vi "gyro -- async pll monitor V2.vi"(8 "pll engine pair IN":T7, 11 "pll monitor event pair IN":T7) -> ()   [LabVIEW 2020]
uses:
  agregator -- action.ctl
  four-corner circle transformation.ctl
  cursor action.ctl
  interpolation state - real.ctl
  publisher action.ctl
  pll internal user event action.ctl
  server talkto message type.ctl
  circle corners.ctl
  lorentzian.ctl
  show-win- control.ctl
  <vilib>/event_ctls.llb/eventvkey.ctl
  server talkback message type.ctl
  server talk-to-back pair.ctl
panel:
  in  "all 3":T1(tab)
  in  "Reset lore :q":bool
  in  "Tab Control":enum32{"PID", "hist", "params"}(tab)=enum."params"
  out "Plot: complex plane":cluster{dbl[], dbl[]}[](graph)=[{[1.788783031557316e-06, 1.7433846913024676e-06, 1.607269314653193e-06, 1.380675694232449e-06, 1.0640013522474786e-06, 6.578018431007985e-07, 1.627897787589622e-07, -4.201664214109396e-07, -1.090044054143964e-06, -1.845667926446343e-06, -2.6857124172833478e-06, -3.6087038031690138e-06, -4.613022843577905e-06, -5.6969076216432555e-06, -6.858456635157808e-06, -8.095632132454864e-06, -9.406263687317083e-06, -1.0788052006641661e-05, -1.2238572964181675e-05, -1.375528185328725e-05, -1.5335517851185776e-05, -1.6976508686969115e-05, -1.8675375505098885e-05, -2.0429137915897256e-05, -2.2234719224163222e-05, -2.4088951826741428e-05, -2.5988582769574486e-05, -2.793027945448972e-05, -2.991063548570884e-05, -3.1926176645823585e-05, -3.397336699075361e-05, -3.604861505299396e-05, -3.814828014226944e-05, -4.026867873254248e-05, -4.240609092416943e-05, -4.455676696986866e-05, -4.671693385305138e-05, -4.888280190697483e-05, -5.105057146310552e-05, -5.321643951702898e-05, -5.5376606400211694e-05, -5.752728244591091e-05, -5.9664694637537876e-05, -6.178509322781091e-05, -6.38847583170864e-05, -6.596000637932674e-05, -6.800719672425677e-05, -7.002273788437151e-05, -7.200309391559062e-05, -7.394479060050587e-05, -7.584442154333893e-05, -7.769865414591714e-05, -7.95042354541831e-05, -8.125799786498148e-05, -8.295686468311124e-05, -8.459785551889458e-05, -8.61780915167931e-05, -8.769480040589868e-05, -8.91453213634387e-05, -9.052710968276327e-05, -9.18377412376255e-05, -9.307491673492255e-05, -9.42364657484371e-05, -9.532035052650245e-05, -9.632466956691135e-05, -9.724766095279701e-05, -9.808770544363402e-05, -9.88433293159364e-05, -9.951320694866943e-05, -0.00010009616314883933, -0.00010059117521318116, -0.00010099737472232784, -0.0001013140490643128, -0.00010154064268473356, -0.00010167675806138284, -0.00010172215640163768, -0.00010167675806138284, -0.00010154064268473356, -0.00010131404906431282, -0.00010099737472232786, -0.00010059117521318118, -0.00010009616314883934, -9.951320694866943e-05, -9.88433293159364e-05, -9.808770544363403e-05, -9.724766095279704e-05, -9.632466956691136e-05, -9.532035052650247e-05, -9.423646574843712e-05, -9.307491673492258e-05, -9.183774123762553e-05, -9.05271096827633e-05, -8.914532136343872e-05, -8.769480040589871e-05, -8.617809151679313e-05, -8.459785551889461e-05, -8.295686468311128e-05, -8.12579978649815e-05, -7.950423545418313e-05, -7.769865414591716e-05, -7.584442154333896e-05, -7.39447906005059e-05, -7.200309391559066e-05, -7.002273788437154e-05, -6.80071967242568e-05, -6.596000637932677e-05, -6.388475831708641e-05, -6.178509322781096e-05, -5.966469463753793e-05, -5.752728244591097e-05, -5.5376606400211735e-05, -5.321643951702903e-05, -5.105057146310557e-05, -4.888280190697487e-05, -4.671693385305141e-05, -4.45567669698687e-05, -4.2406090924169466e-05, -4.02686787325425e-05, -3.814828014226947e-05, -3.604861505299398e-05, -3.3973366990753624e-05, -3.192617664582364e-05, -2.9910635485708896e-05, -2.7930279454489773e-05, -2.5988582769574527e-05, -2.4088951826741472e-05, -2.223471922416326e-05, -2.042913791589729e-05, -1.8675375505098912e-05, -1.6976508686969142e-05, -1.5335517851185796e-05, -1.375528185328727e-05, -1.2238572964181688e-05, -1.0788052006641675e-05, -9.406263687317096e-06, -8.09563213245487e-06, -6.858456635157842e-06, -5.696907621643283e-06, -4.613022843577932e-06, -3.608703803169034e-06, -2.685712417283368e-06, -1.8456679264463634e-06, -1.0900440541439775e-06, -4.2016642141095315e-07, 1.6278977875895542e-07, 6.578018431007917e-07, 1.0640013522474786e-06, 1.3806756942324422e-06, 1.607269314653193e-06, 1.7433846913024676e-06], [0.00010355923614313292, 0.00010572653027157724, 0.00010789002222966876, 0.00011004591651735351, 0.00011219043096347307, 0.00011431980336097804, 0.00011643029806711761, 0.00011851821255702628, 0.00012057988391921064, 0.00012261169528154077, 0.00012461008215647302, 0.00012657153869437233, 0.00012849262383396383, 0.00013036996733912354, 0.0001322002757114178, 0.00013398033796801863, 0.00013570703127485878, 0.00013737732642514367, 0.00013898829315360961, 0.00014053710527720475, 0.00014202104565317432, 0.00014343751094585263, 0.0001447840161937981, 0.0001460581991692603, 0.00014725782452233005, 0.00014838078770250255, 0.00014942511865077436, 0.00015038898525579616, 0.00015127069656801869, 0.00015206870576619277, 0.00015278161287101945, 0.00015340816720118942, 0.00015394726956750299, 0.0001543979742012214, 0.0001547594904132666, 0.00015503118398135874, 0.00015521257826265722, 0.00015530335502995444, 0.00015530335502995444, 0.00015521257826265722, 0.00015503118398135874, 0.00015475949041326664, 0.0001543979742012214, 0.00015394726956750299, 0.00015340816720118942, 0.00015278161287101945, 0.00015206870576619277, 0.0001512706965680187, 0.0001503889852557962, 0.00014942511865077439, 0.00014838078770250258, 0.00014725782452233005, 0.00014605819916926034, 0.0001447840161937981, 0.00014343751094585263, 0.00014202104565317434, 0.00014053710527720475, 0.00013898829315360964, 0.0001373773264251437, 0.00013570703127485878, 0.00013398033796801863, 0.00013220027571141782, 0.00013036996733912354, 0.00012849262383396383, 0.00012657153869437236, 0.00012461008215647305, 0.0001226116952815408, 0.00012057988391921064, 0.00011851821255702631, 0.00011643029806711764, 0.00011431980336097807, 0.00011219043096347309, 0.00011004591651735353, 0.00010789002222966877, 0.00010572653027157724, 0.00010355923614313295, 0.00010139194201468863, 9.92284500565971e-05, 9.707255576891236e-05, 9.492804132279279e-05, 9.279866892528782e-05, 9.068817421914825e-05, 8.860025972923959e-05, 8.653858836705524e-05, 8.45067770047251e-05, 8.250839012979284e-05, 8.054693359189351e-05, 7.862584845230203e-05, 7.674850494714233e-05, 7.491819657484808e-05, 7.313813431824723e-05, 7.141144101140709e-05, 6.97411458611222e-05, 6.813017913265623e-05, 6.658136700906111e-05, 6.509742663309153e-05, 6.368096134041324e-05, 6.233445609246777e-05, 6.106027311700553e-05, 5.9860647763935806e-05, 5.87376845837633e-05, 5.769335363549149e-05, 5.6729487030469677e-05, 5.584777571824716e-05, 5.5049766520073076e-05, 5.433685941524639e-05, 5.371030508507641e-05, 5.317120271876287e-05, 5.2720498085044465e-05, 5.235898187299923e-05, 5.2087288304907106e-05, 5.1905894023608635e-05, 5.181511725631141e-05, 5.18151172563114e-05, 5.1905894023608635e-05, 5.20872883049071e-05, 5.2358981872999216e-05, 5.272049808504446e-05, 5.3171202718762854e-05, 5.37103050850764e-05, 5.433685941524638e-05, 5.5049766520073056e-05, 5.584777571824713e-05, 5.672948703046965e-05, 5.769335363549145e-05, 5.8737684583763264e-05, 5.986064776393577e-05, 6.10602731170055e-05, 6.233445609246772e-05, 6.368096134041321e-05, 6.50974266330915e-05, 6.658136700906109e-05, 6.81301791326562e-05, 6.974114586112215e-05, 7.141144101140706e-05, 7.31381343182472e-05, 7.491819657484801e-05, 7.674850494714228e-05, 7.862584845230197e-05, 8.054693359189346e-05, 8.250839012979277e-05, 8.450677700472503e-05, 8.653858836705518e-05, 8.860025972923954e-05, 9.06881742191482e-05, 9.279866892528778e-05, 9.492804132279275e-05, 9.70725557689123e-05, 9.922845005659706e-05, 0.00010139194201468859]}, {[1.679879022748994e-06, -3.4847775480299235e-06, -8.649434118808841e-06, -1.3814090689587757e-05, -1.8978747260366676e-05, -2.4143403831145596e-05, -2.9308060401924508e-05, -3.447271697270343e-05, -3.963737354348235e-05, -4.4802030114261266e-05, -4.9966686685040185e-05, -5.51313432558191e-05, -6.029599982659801e-05, -6.546065639737694e-05, -7.062531296815585e-05, -7.578996953893478e-05, -8.095462610971369e-05, -8.61192826804926e-05, -9.128393925127153e-05, -9.644859582205044e-05], [0.00010691496202238116, 0.00010657938943445635, 0.00010624381684653152, 0.00010590824425860668, 0.00010557267167068187, 0.00010523709908275705, 0.00010490152649483222, 0.00010456595390690739, 0.00010423038131898257, 0.00010389480873105775, 0.00010355923614313292, 0.00010322366355520809, 0.00010288809096728327, 0.00010255251837935846, 0.00010221694579143363, 0.0001018813732035088, 0.00010154580061558398, 0.00010121022802765916, 0.00010087465543973433, 0.0001005390828518095]}, {[-4.6610960805791945e-05, -4.694653339371677e-05, -4.728210598164159e-05, -4.761767856956642e-05, -4.795325115749124e-05, -4.8288823745416065e-05, -4.862439633334089e-05, -4.895996892126571e-05, -4.929554150919054e-05, -4.963111409711536e-05, -4.9966686685040185e-05, -5.0302259272965016e-05, -5.0637831860889833e-05, -5.0973404448814664e-05, -5.130897703673949e-05, -5.164454962466431e-05, -5.1980122212589136e-05, -5.231569480051396e-05, -5.2651267388438784e-05, -5.298683997636361e-05], [5.191267043534376e-05, 5.7077327006122676e-05, 6.22419835769016e-05, 6.740664014768051e-05, 7.257129671845942e-05, 7.773595328923835e-05, 8.290060986001726e-05, 8.806526643079617e-05, 9.322992300157508e-05, 9.839457957235401e-05, 0.00010355923614313292, 0.00010872389271391185, 0.00011388854928469076, 0.00011905320585546967, 0.0001242178624262486, 0.00012938251899702753, 0.00013454717556780644, 0.00013971183213858535, 0.00014487648870936426, 0.00015004114528014318]}, {[8.391330781245461e-06, 7.720185605395813e-06, 7.049040429546165e-06, 6.377895253696517e-06, 5.706750077846869e-06, 5.035604901997221e-06, 4.364459726147573e-06, 3.6933145502979247e-06, 3.0221693744482766e-06, 2.3510241985986286e-06, 1.6798790227489805e-06, 1.0087338468993325e-06, 3.3758867104968446e-07, -3.335565047999636e-07, -1.0047016806496116e-06, -1.6758468564992597e-06, -2.3469920323489077e-06, -3.0181372081985558e-06, -3.689282384048204e-06, -4.360427559897852e-06], [3.6218306068028043e-06, 1.395114374836064e-05, 2.4280456889918475e-05, 3.4609770031476307e-05, 4.4939083173034145e-05, 5.5268396314591984e-05, 6.559770945614981e-05, 7.592702259770765e-05, 8.625633573926549e-05, 9.658564888082332e-05, 0.00010691496202238116, 0.00011724427516393899, 0.0001275735883054968, 0.00013790290144705467, 0.0001482322145886125, 0.00015856152773017034, 0.00016889084087172817, 0.000179220154013286, 0.00018954946715484384, 0.00019987878029640167]}]
  out "Plot: complex- hist":cluster{dbl[], dbl[]}[](graph)=[{array[1000 elements], array[1000 elements]}, {[1.788783031557316e-06, 1.7433846913024676e-06, 1.607269314653193e-06, 1.380675694232449e-06, 1.0640013522474786e-06, 6.578018431007985e-07, 1.627897787589622e-07, -4.201664214109396e-07, -1.090044054143964e-06, -1.845667926446343e-06, -2.6857124172833478e-06, -3.6087038031690138e-06, -4.613022843577905e-06, -5.6969076216432555e-06, -6.858456635157808e-06, -8.095632132454864e-06, -9.406263687317083e-06, -1.0788052006641661e-05, -1.2238572964181675e-05, -1.375528185328725e-05, -1.5335517851185776e-05, -1.6976508686969115e-05, -1.8675375505098885e-05, -2.0429137915897256e-05, -2.2234719224163222e-05, -2.4088951826741428e-05, -2.5988582769574486e-05, -2.793027945448972e-05, -2.991063548570884e-05, -3.1926176645823585e-05, -3.397336699075361e-05, -3.604861505299396e-05, -3.814828014226944e-05, -4.026867873254248e-05, -4.240609092416943e-05, -4.455676696986866e-05, -4.671693385305138e-05, -4.888280190697483e-05, -5.105057146310552e-05, -5.321643951702898e-05, -5.5376606400211694e-05, -5.752728244591091e-05, -5.9664694637537876e-05, -6.178509322781091e-05, -6.38847583170864e-05, -6.596000637932674e-05, -6.800719672425677e-05, -7.002273788437151e-05, -7.200309391559062e-05, -7.394479060050587e-05, -7.584442154333893e-05, -7.769865414591714e-05, -7.95042354541831e-05, -8.125799786498148e-05, -8.295686468311124e-05, -8.459785551889458e-05, -8.61780915167931e-05, -8.769480040589868e-05, -8.91453213634387e-05, -9.052710968276327e-05, -9.18377412376255e-05, -9.307491673492255e-05, -9.42364657484371e-05, -9.532035052650245e-05, -9.632466956691135e-05, -9.724766095279701e-05, -9.808770544363402e-05, -9.88433293159364e-05, -9.951320694866943e-05, -0.00010009616314883933, -0.00010059117521318116, -0.00010099737472232784, -0.0001013140490643128, -0.00010154064268473356, -0.00010167675806138284, -0.00010172215640163768, -0.00010167675806138284, -0.00010154064268473356, -0.00010131404906431282, -0.00010099737472232786, -0.00010059117521318118, -0.00010009616314883934, -9.951320694866943e-05, -9.88433293159364e-05, -9.808770544363403e-05, -9.724766095279704e-05, -9.632466956691136e-05, -9.532035052650247e-05, -9.423646574843712e-05, -9.307491673492258e-05, -9.183774123762553e-05, -9.05271096827633e-05, -8.914532136343872e-05, -8.769480040589871e-05, -8.617809151679313e-05, -8.459785551889461e-05, -8.295686468311128e-05, -8.12579978649815e-05, -7.950423545418313e-05, -7.769865414591716e-05, -7.584442154333896e-05, -7.39447906005059e-05, -7.200309391559066e-05, -7.002273788437154e-05, -6.80071967242568e-05, -6.596000637932677e-05, -6.388475831708641e-05, -6.178509322781096e-05, -5.966469463753793e-05, -5.752728244591097e-05, -5.5376606400211735e-05, -5.321643951702903e-05, -5.105057146310557e-05, -4.888280190697487e-05, -4.671693385305141e-05, -4.45567669698687e-05, -4.2406090924169466e-05, -4.02686787325425e-05, -3.814828014226947e-05, -3.604861505299398e-05, -3.3973366990753624e-05, -3.192617664582364e-05, -2.9910635485708896e-05, -2.7930279454489773e-05, -2.5988582769574527e-05, -2.4088951826741472e-05, -2.223471922416326e-05, -2.042913791589729e-05, -1.8675375505098912e-05, -1.6976508686969142e-05, -1.5335517851185796e-05, -1.375528185328727e-05, -1.2238572964181688e-05, -1.0788052006641675e-05, -9.406263687317096e-06, -8.09563213245487e-06, -6.858456635157842e-06, -5.696907621643283e-06, -4.613022843577932e-06, -3.608703803169034e-06, -2.685712417283368e-06, -1.8456679264463634e-06, -1.0900440541439775e-06, -4.2016642141095315e-07, 1.6278977875895542e-07, 6.578018431007917e-07, 1.0640013522474786e-06, 1.3806756942324422e-06, 1.607269314653193e-06, 1.7433846913024676e-06], [0.00010355923614313292, 0.00010572653027157724, 0.00010789002222966876, 0.00011004591651735351, 0.00011219043096347307, 0.00011431980336097804, 0.00011643029806711761, 0.00011851821255702628, 0.00012057988391921064, 0.00012261169528154077, 0.00012461008215647302, 0.00012657153869437233, 0.00012849262383396383, 0.00013036996733912354, 0.0001322002757114178, 0.00013398033796801863, 0.00013570703127485878, 0.00013737732642514367, 0.00013898829315360961, 0.00014053710527720475, 0.00014202104565317432, 0.00014343751094585263, 0.0001447840161937981, 0.0001460581991692603, 0.00014725782452233005, 0.00014838078770250255, 0.00014942511865077436, 0.00015038898525579616, 0.00015127069656801869, 0.00015206870576619277, 0.00015278161287101945, 0.00015340816720118942, 0.00015394726956750299, 0.0001543979742012214, 0.0001547594904132666, 0.00015503118398135874, 0.00015521257826265722, 0.00015530335502995444, 0.00015530335502995444, 0.00015521257826265722, 0.00015503118398135874, 0.00015475949041326664, 0.0001543979742012214, 0.00015394726956750299, 0.00015340816720118942, 0.00015278161287101945, 0.00015206870576619277, 0.0001512706965680187, 0.0001503889852557962, 0.00014942511865077439, 0.00014838078770250258, 0.00014725782452233005, 0.00014605819916926034, 0.0001447840161937981, 0.00014343751094585263, 0.00014202104565317434, 0.00014053710527720475, 0.00013898829315360964, 0.0001373773264251437, 0.00013570703127485878, 0.00013398033796801863, 0.00013220027571141782, 0.00013036996733912354, 0.00012849262383396383, 0.00012657153869437236, 0.00012461008215647305, 0.0001226116952815408, 0.00012057988391921064, 0.00011851821255702631, 0.00011643029806711764, 0.00011431980336097807, 0.00011219043096347309, 0.00011004591651735353, 0.00010789002222966877, 0.00010572653027157724, 0.00010355923614313295, 0.00010139194201468863, 9.92284500565971e-05, 9.707255576891236e-05, 9.492804132279279e-05, 9.279866892528782e-05, 9.068817421914825e-05, 8.860025972923959e-05, 8.653858836705524e-05, 8.45067770047251e-05, 8.250839012979284e-05, 8.054693359189351e-05, 7.862584845230203e-05, 7.674850494714233e-05, 7.491819657484808e-05, 7.313813431824723e-05, 7.141144101140709e-05, 6.97411458611222e-05, 6.813017913265623e-05, 6.658136700906111e-05, 6.509742663309153e-05, 6.368096134041324e-05, 6.233445609246777e-05, 6.106027311700553e-05, 5.9860647763935806e-05, 5.87376845837633e-05, 5.769335363549149e-05, 5.6729487030469677e-05, 5.584777571824716e-05, 5.5049766520073076e-05, 5.433685941524639e-05, 5.371030508507641e-05, 5.317120271876287e-05, 5.2720498085044465e-05, 5.235898187299923e-05, 5.2087288304907106e-05, 5.1905894023608635e-05, 5.181511725631141e-05, 5.18151172563114e-05, 5.1905894023608635e-05, 5.20872883049071e-05, 5.2358981872999216e-05, 5.272049808504446e-05, 5.3171202718762854e-05, 5.37103050850764e-05, 5.433685941524638e-05, 5.5049766520073056e-05, 5.584777571824713e-05, 5.672948703046965e-05, 5.769335363549145e-05, 5.8737684583763264e-05, 5.986064776393577e-05, 6.10602731170055e-05, 6.233445609246772e-05, 6.368096134041321e-05, 6.50974266330915e-05, 6.658136700906109e-05, 6.81301791326562e-05, 6.974114586112215e-05, 7.141144101140706e-05, 7.31381343182472e-05, 7.491819657484801e-05, 7.674850494714228e-05, 7.862584845230197e-05, 8.054693359189346e-05, 8.250839012979277e-05, 8.450677700472503e-05, 8.653858836705518e-05, 8.860025972923954e-05, 9.06881742191482e-05, 9.279866892528778e-05, 9.492804132279275e-05, 9.70725557689123e-05, 9.922845005659706e-05, 0.00010139194201468859]}, {[1.679879022748994e-06, -3.4847775480299235e-06, -8.649434118808841e-06, -1.3814090689587757e-05, -1.8978747260366676e-05, -2.4143403831145596e-05, -2.9308060401924508e-05, -3.447271697270343e-05, -3.963737354348235e-05, -4.4802030114261266e-05, -4.9966686685040185e-05, -5.51313432558191e-05, -6.029599982659801e-05, -6.546065639737694e-05, -7.062531296815585e-05, -7.578996953893478e-05, -8.095462610971369e-05, -8.61192826804926e-05, -9.128393925127153e-05, -9.644859582205044e-05], [0.00010691496202238116, 0.00010657938943445635, 0.00010624381684653152, 0.00010590824425860668, 0.00010557267167068187, 0.00010523709908275705, 0.00010490152649483222, 0.00010456595390690739, 0.00010423038131898257, 0.00010389480873105775, 0.00010355923614313292, 0.00010322366355520809, 0.00010288809096728327, 0.00010255251837935846, 0.00010221694579143363, 0.0001018813732035088, 0.00010154580061558398, 0.00010121022802765916, 0.00010087465543973433, 0.0001005390828518095]}, {[-4.6610960805791945e-05, -4.694653339371677e-05, -4.728210598164159e-05, -4.761767856956642e-05, -4.795325115749124e-05, -4.8288823745416065e-05, -4.862439633334089e-05, -4.895996892126571e-05, -4.929554150919054e-05, -4.963111409711536e-05, -4.9966686685040185e-05, -5.0302259272965016e-05, -5.0637831860889833e-05, -5.0973404448814664e-05, -5.130897703673949e-05, -5.164454962466431e-05, -5.1980122212589136e-05, -5.231569480051396e-05, -5.2651267388438784e-05, -5.298683997636361e-05], [5.191267043534376e-05, 5.7077327006122676e-05, 6.22419835769016e-05, 6.740664014768051e-05, 7.257129671845942e-05, 7.773595328923835e-05, 8.290060986001726e-05, 8.806526643079617e-05, 9.322992300157508e-05, 9.839457957235401e-05, 0.00010355923614313292, 0.00010872389271391185, 0.00011388854928469076, 0.00011905320585546967, 0.0001242178624262486, 0.00012938251899702753, 0.00013454717556780644, 0.00013971183213858535, 0.00014487648870936426, 0.00015004114528014318]}, {[8.391330781245461e-06, 7.720185605395813e-06, 7.049040429546165e-06, 6.377895253696517e-06, 5.706750077846869e-06, 5.035604901997221e-06, 4.364459726147573e-06, 3.6933145502979247e-06, 3.0221693744482766e-06, 2.3510241985986286e-06, 1.6798790227489805e-06, 1.0087338468993325e-06, 3.3758867104968446e-07, -3.335565047999636e-07, -1.0047016806496116e-06, -1.6758468564992597e-06, -2.3469920323489077e-06, -3.0181372081985558e-06, -3.689282384048204e-06, -4.360427559897852e-06], [3.6218306068028043e-06, 1.395114374836064e-05, 2.4280456889918475e-05, 3.4609770031476307e-05, 4.4939083173034145e-05, 5.5268396314591984e-05, 6.559770945614981e-05, 7.592702259770765e-05, 8.625633573926549e-05, 9.658564888082332e-05, 0.00010691496202238116, 0.00011724427516393899, 0.0001275735883054968, 0.00013790290144705467, 0.0001482322145886125, 0.00015856152773017034, 0.00016889084087172817, 0.000179220154013286, 0.00018954946715484384, 0.00019987878029640167]}, {[nan, nan, nan, nan, nan, nan, nan, nan, nan, nan, nan, nan, nan, nan, nan, nan, nan, nan, nan, nan], [nan, nan, nan, nan, nan, nan, nan, nan, nan, nan, nan, nan, nan, nan, nan, nan, nan, nan, nan, nan]}]
  in  "dt (sec)":dbl=0.001 format="%#_10f"
  in  "plot hist time (sec)":dbl=1.0 format="%#_10f"
  out "G (Hz)":dbl=inf format="%#.4f"
  in  "Reset freq :r":bool
  in  "lorentzian":T2={"A (VHz)"=0.0013462087701026876, "f (Hz)"=46382.17969574165, "G (Hz)"=26.010946813433538, "phi(rad)"=-1.5059127195190136, "Q"=1783.1792140602604, "Norm  Ampl"=nan, "bg (V)"=1.6798790227489873e-06+0.00010691496202238116i, "4corners"={"z (-pi/2)"=-4.6610960805791945e-05+5.191267043534375e-05i, "z(inf)"=1.6798790227489873e-06+0.00010691496202238116i, "z (pi/2)"=-5.332241256428843e-05+0.0001552058018509221i, "z center"=-4.9966686685040185e-05+0.00010355923614313292i, "z(0)"=-0.00010161325239282936+0.00010020351026388468i, "radius"=5.17554697165975e-05}} {"bg (V)" format="%#9_9f"; "Q" format="%#9_9f"; "phi(rad)" format="%#9_9f"; "G (Hz)" format="%#9_9f"; "f (Hz)" format="%#9_9f"}
  in  "Toggle PLL :@":bool
  out "f (Hz)":dbl=6.94898403792542e-310 format="%#.11f"
  in  "PLL is ON":bool
  in  "publish delay":u32=30
  out "VKey":T4=enum."Cmd"
  out "Char":i16
  in  "lorentzian -- basic":T2={"A (VHz)"=1.0, "f (Hz)"=1000.0, "G (Hz)"=3.0, "phi(rad)"=0.0, "Q"=300.0, "Norm  Ampl"=nan, "bg (V)"=0.0+0.0i, "4corners"={"z (-pi/2)"=9.277908004825974e-07+0.0007240755403629966i, "z(inf)"=2.6527949823343002e-05+0.0007477540585896028i, "z (pi/2)"=2.8494315967368497e-06+0.0007733542176124632i, "z center"=1.8886111986097237e-06+0.0007487148789877299i, "z(0)"=-2.2750727426123552e-05+0.000749675699385857i, "radius"=2.4658065287076567e-05}} {"bg (V)" format="%#9_9f"; "Q" format="%#9_9f"; "phi(rad)" format="%#9_9f"; "G (Hz)" format="%#9_9f"; "f (Hz)" format="%#9_9f"}
  in  "save lor for later":bool
  in  "reset from basic":bool
  out "zi out Im (V)":dbl=8e-323 format="%#.8f"
  out "zi out Re (V)":dbl=1e-323 format="%#.8f"
  out "publish message":T5={"freq (Hz)"=6.94898403792542e-310, "gamma (Hz)"=inf, "Voltage (V)"=1e-323+8e-323i}
  out "is publish loop stoped?":bool=TRUE
  out "window":T6={"cen (Hz)"=45496.74569300777, "win (Hz)"=29.962105514646385, "left (Hz)"=45481.76464025045, "right (Hz)"=45511.72674576509}
  in  "lorentzian -- hist":T2={"A (VHz)"=0.0013462087701026876, "f (Hz)"=46382.17969574165, "G (Hz)"=26.010946813433538, "phi(rad)"=-1.5059127195190136, "Q"=1783.1792140602604, "Norm  Ampl"=nan, "bg (V)"=1.6798790227489873e-06+0.00010691496202238116i, "4corners"={"z (-pi/2)"=-4.6610960805791945e-05+5.191267043534375e-05i, "z(inf)"=1.6798790227489873e-06+0.00010691496202238116i, "z (pi/2)"=-5.332241256428843e-05+0.0001552058018509221i, "z center"=-4.9966686685040185e-05+0.00010355923614313292i, "z(0)"=-0.00010161325239282936+0.00010020351026388468i, "radius"=5.17554697165975e-05}} {"bg (V)" format="%#9_9f"; "Q" format="%#9_9f"; "phi(rad)" format="%#9_9f"; "G (Hz)" format="%#9_9f"; "f (Hz)" format="%#9_9f"}
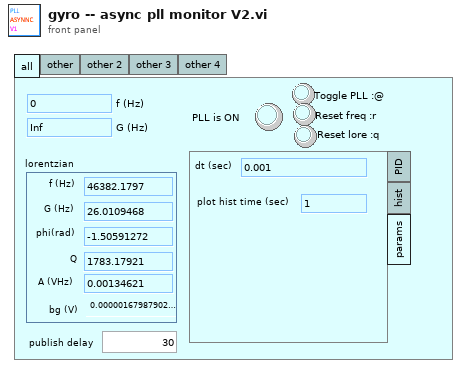
[diagram p1: front panel]
types:
  T1 = enum32{"all", "other", "other 2", "other 3", "other 4"}
  T2 = typedef "lorentzian.ctl" = cluster{"A (VHz)":dbl, "f (Hz)":dbl, "G (Hz)":dbl, "phi(rad)":dbl, "Q":dbl, "Norm  Ampl":dbl, "bg (V)":cdb, "4corners":T3}
  T3 = typedef "circle corners.ctl" = cluster{"z (-pi/2)":cdb, "z(inf)":cdb, "z (pi/2)":cdb, "z center":cdb, "z(0)":cdb, "radius":dbl}
  T4 = typedef "eventvkey.ctl" = enum16{"ASCII", "Enter", "Return", "Shift", "Ctrl", "Alt", "Cmd", "Opt", "Caps", "NumLock", "Clear", "Break", "Up", "Down", "Left", "Right", "Insert", "Delete", "Home", "End", "PageUp", "PageDown", "Escape", "Help", "Pause", "ScrollLock", "F1", "F2", "F3", "F4", "F5", "F6", "F7", "F8", "F9", "F10", "F11", "F12", "F13", "F14", "F15", "F16", "F17", "F18", "F19", "F20", "F21", "F22", "F23", "F24", "Play", "VolumeUp", "VolumeDown", "Mute", "Two Byte Char"}
  T5 = cluster{"freq (Hz)":dbl, "gamma (Hz)":dbl, "Voltage (V)":cdb}
  T6 = typedef "show-win- control.ctl" = cluster{"cen (Hz)":dbl, "win (Hz)":dbl, "left (Hz)":dbl, "right (Hz)":dbl}
  T7 = typedef "server talk-to-back pair.ctl" = cluster{"talkback event":refnum<user-event>, "talkto event":refnum<user-event>}
  T8 = typedef "pll internal user event action.ctl" = enum16{"gear pll engine", "start pll async", "stop pll async", "toggle pll async", "gear sweeper", "start sweeper", "stop sweeper", "toggle sweeper", "accept frequency", "reset lorentzian", "accept lorentzian", "update cursors", "pause pll", "unpause pll", "void", "exit", "gear sweeper monitor", "gear sweeper engine", "gear fitter", "gear sourcer", "gear pll monitor"}
  T9 = typedef "interpolation state - real.ctl" = cluster{"requested size":i32, "Array":dbl[], "actual number of elements":i32}
  T10 = typedef "agregator -- action.ctl" = enum16{"append", "interpolate", "empty!", "force", "init", "scale", "read last"}
  T11 = typedef "publisher action.ctl" = enum16{"set", "get", "init", "check"}
  T12 = typedef "four-corner circle transformation.ctl" = enum16{"z(c) z(inf)", "z(c) z(zero)", "fix phase", "calculate lorentzian", "z(0) z(+-pi/2)", "shift to zcenter", "to  canonical", "get canonical phase", "get4corners", "update lorentzian -- from z0", "fake gamma normal", "fake gamma heat", "calculate complex slope", "get f0 given f and phi"}
  T13 = typedef "interpolation state - complex.ctl" = cluster{"requested size":i32, "Array":cdb[], "actual number of elements":i32}
  T14 = typedef "server talkto message type.ctl" = cluster{"message":enum16{"stop", "start", "update pars", "update request", "new", "launch", "exit", "get", "reset", "pause", "unpause"}}
  T15 = typedef "cursor action.ctl" = enum16{"range", "read", "write", "check", "zoom out", "smart zoom out", "zoom to aspect ratio 1", "zoom to win", "zoom out 20%", "zoom in 20%", "-empty", "smart zoom out&aspect", "move range left 20%", "move range right 20%", "move range up 20%", "move range down 20%", "zoom to X win", "zoom to Y win", "zoom out X", "zoom out Y", "zoom in X", "zoom in Y", "check plot scale"}
  T16 = typedef "pll talkback data type.ctl" = cluster{"freq (Hz)":dbl, "gamma (Hz)":dbl, "Voltage (V)":cdb, "overlimit ?":bool, "running lorentzian out":T2, "static lorentzian out":T2}
  T17 = enum16{"stop", "start", "update pars", "update request", "new", "launch", "exit", "get", "reset", "pause", "unpause"}
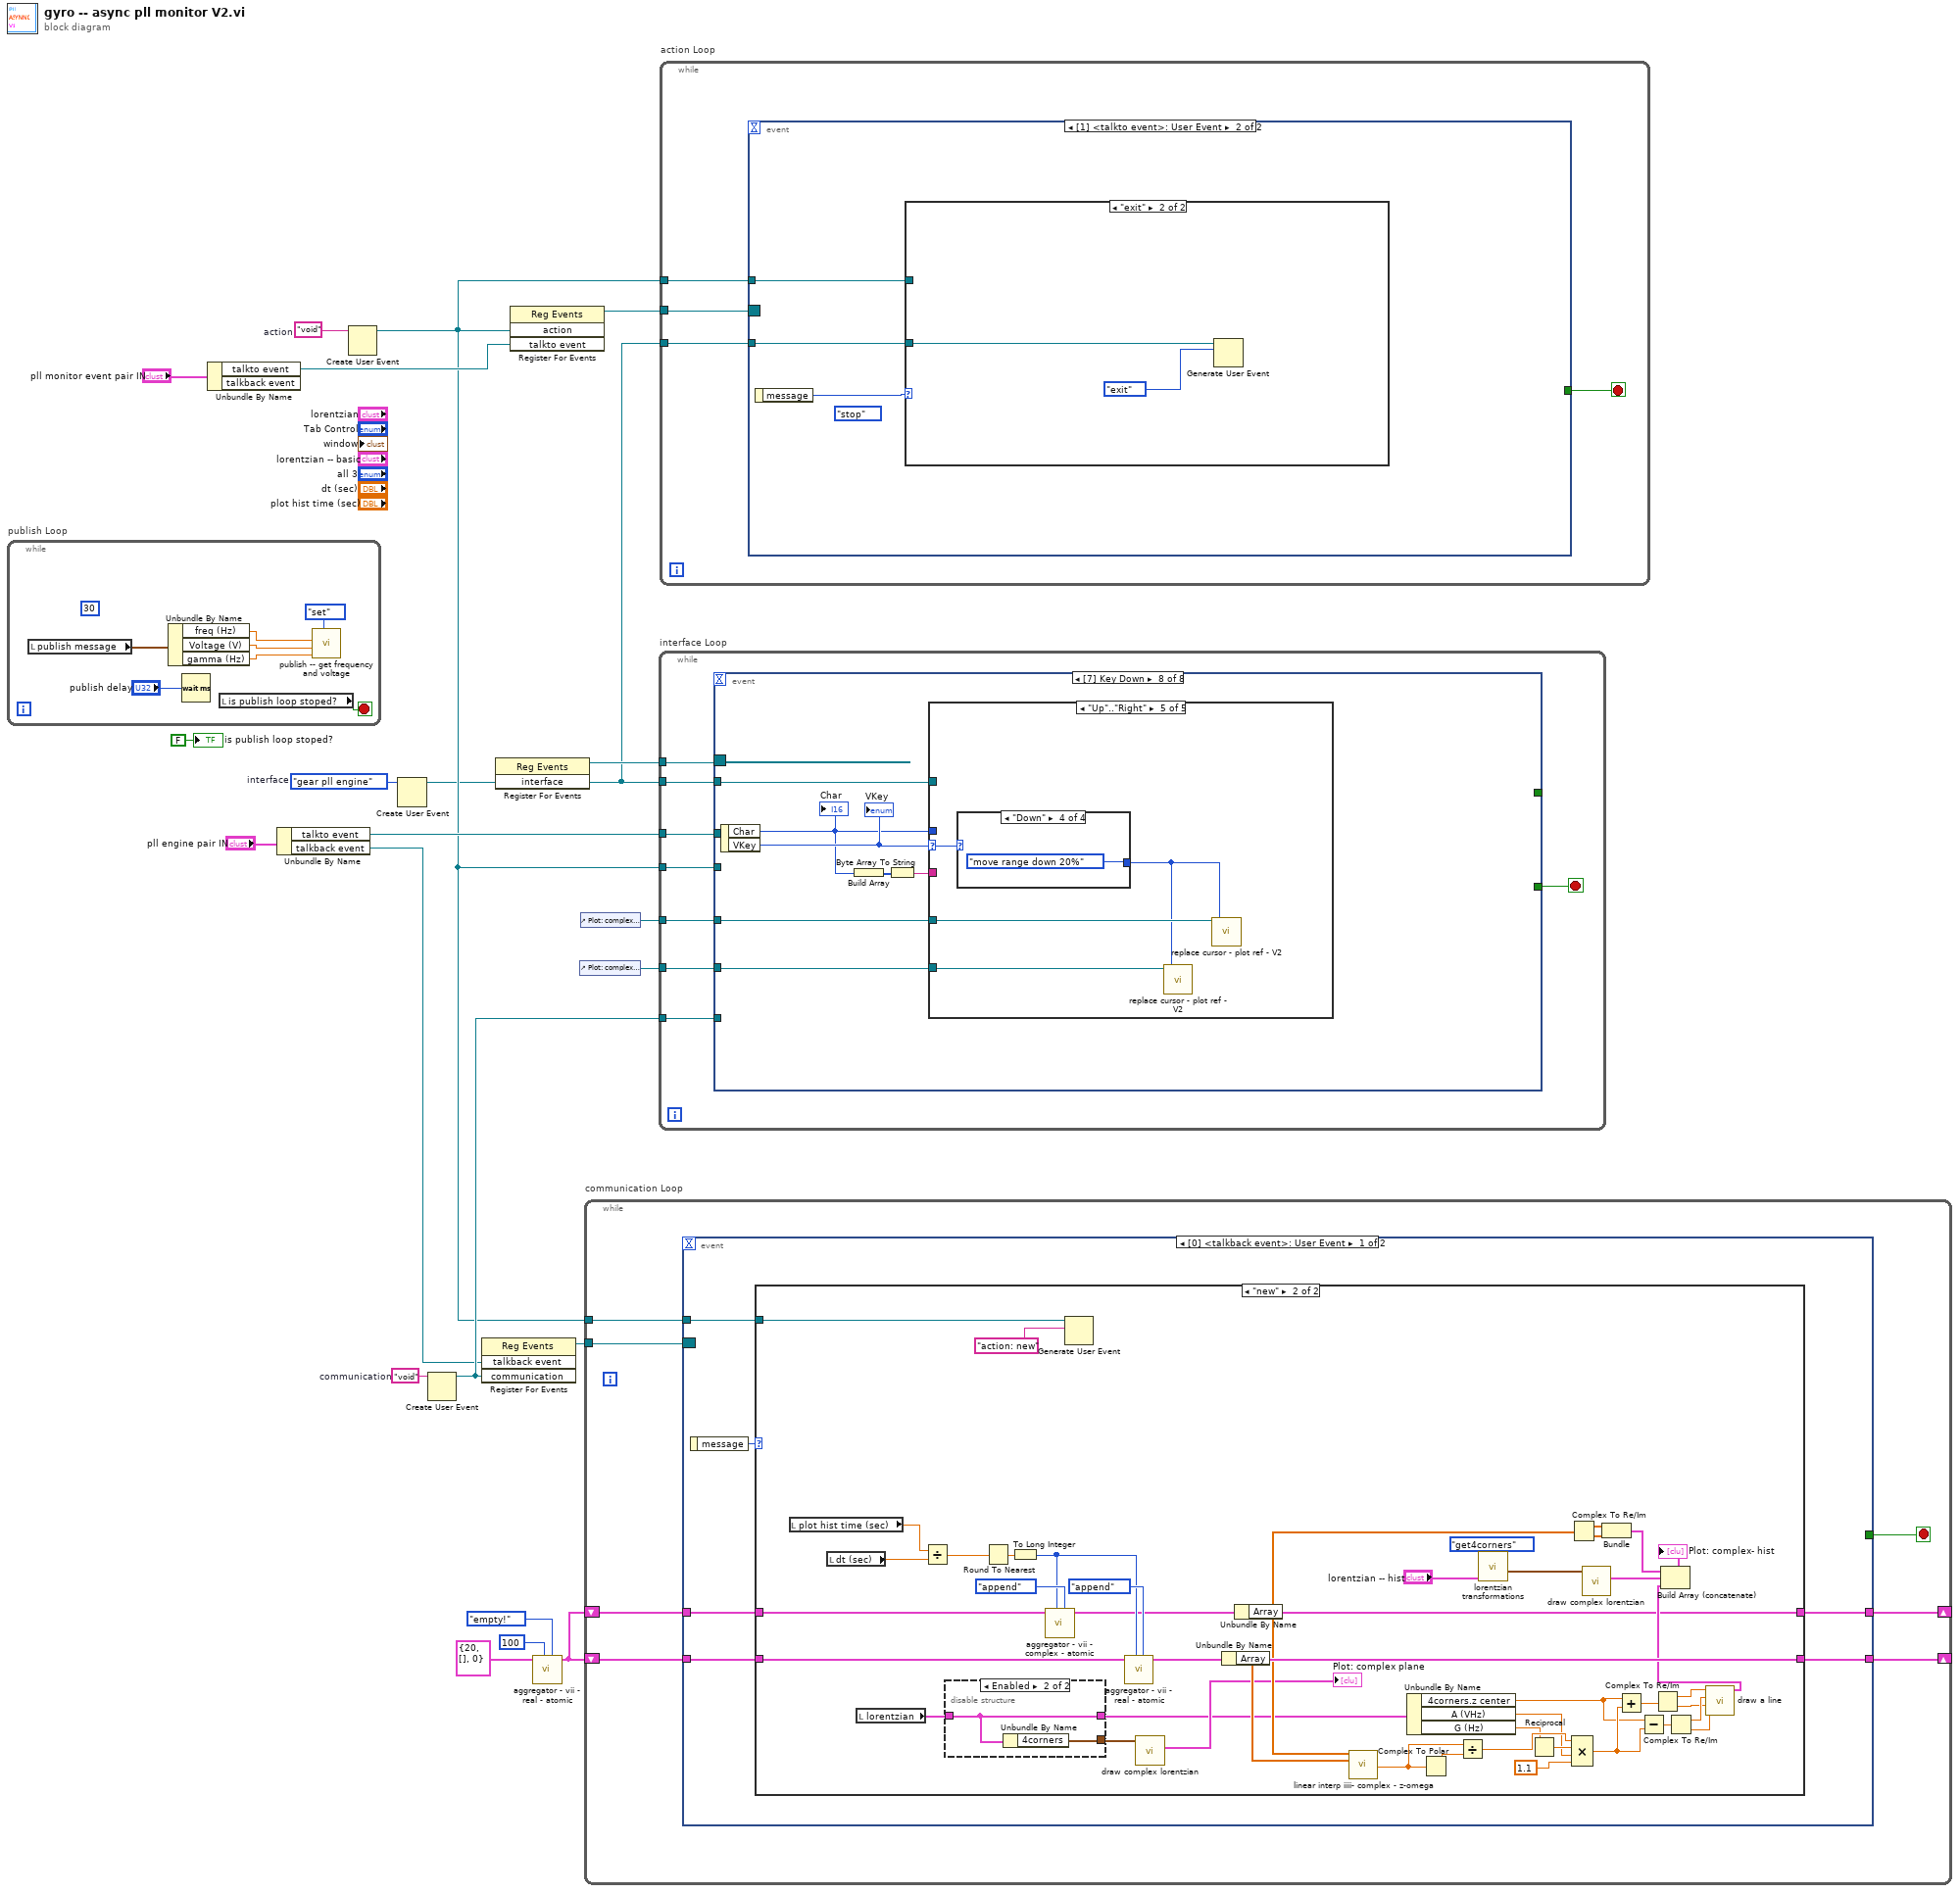
[diagram p0: block diagram]
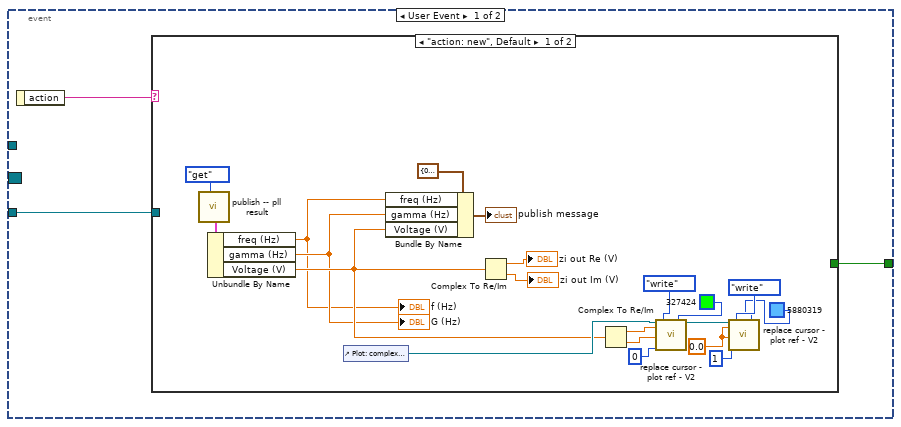
[diagram p2: hidden frame]
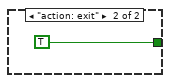
[diagram p3: hidden frame]
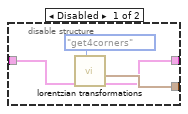
[diagram p6: hidden frame]
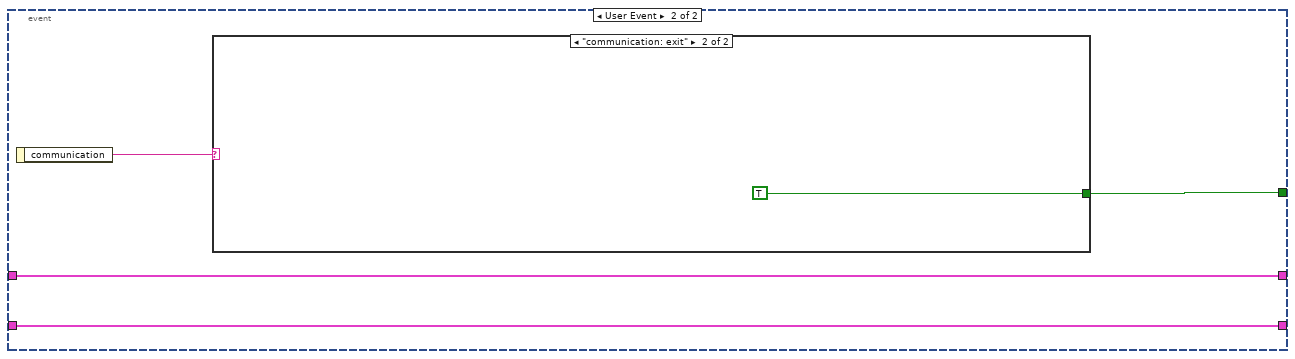
[diagram p7: hidden frame]
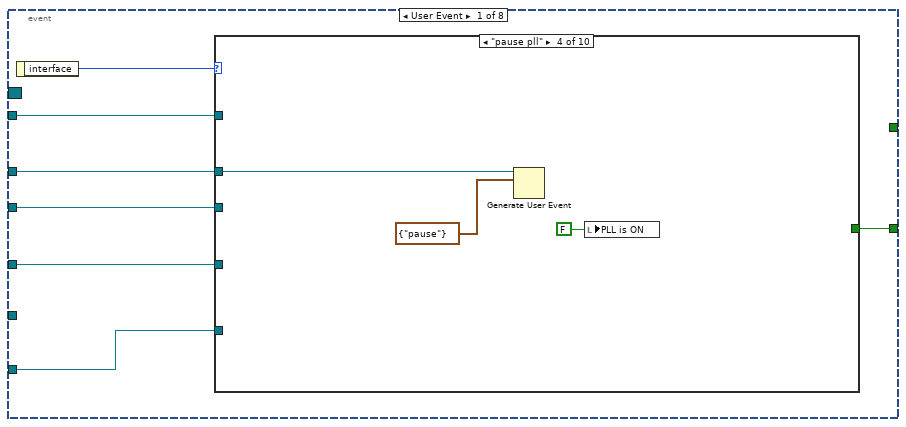
[diagram p9: hidden frame]
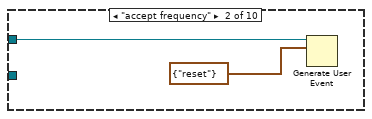
[diagram p11: hidden frame]
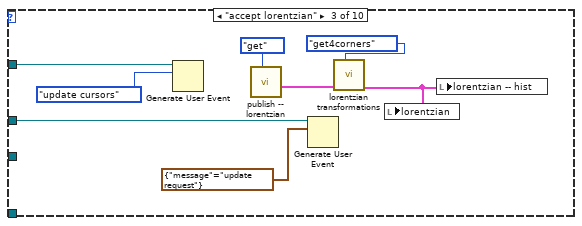
[diagram p12: hidden frame]
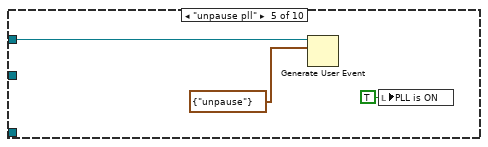
[diagram p13: hidden frame]
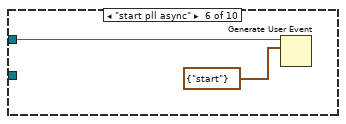
[diagram p14: hidden frame]
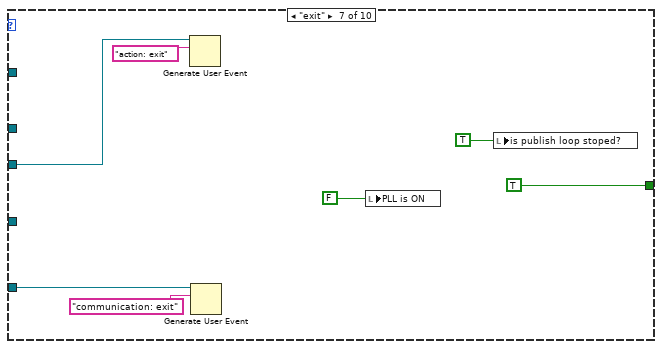
[diagram p15: hidden frame]
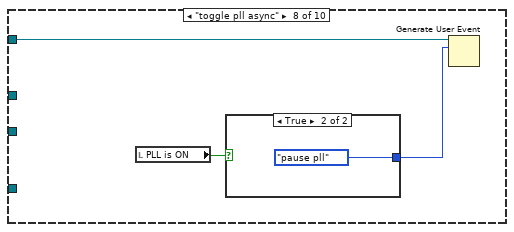
[diagram p16: hidden frame]
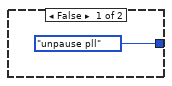
[diagram p17: hidden frame]
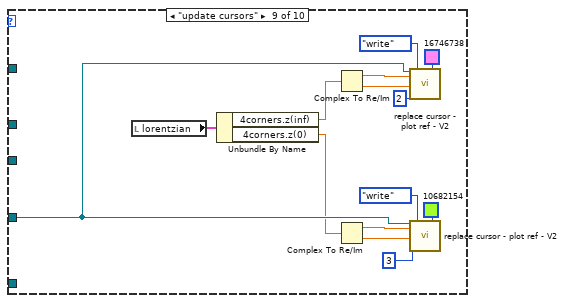
[diagram p18: hidden frame]
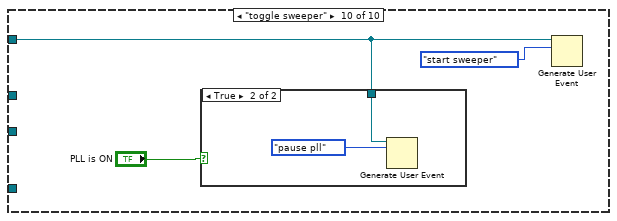
[diagram p19: hidden frame]
diagram:
  w9 = "void"  # communication
  w11 = "void"  # action
  w13 = pll_internal_user_event_action."gear pll engine"  # interface
  n1 = while "publish Loop" {
    stop <- w23 stop-if-true
    (unwired) u32 30 ("milliseconds to wait")
    n2 = local read "publish message"() -> (w27:T5)
    n3 = Unbundle By Name(w27) -> ("freq (Hz)"=w26:dbl, "Voltage (V)"=w25:cdb, "gamma (Hz)"=w24:dbl)
    n4 = Wait (ms)(milliseconds to wait="publish delay") -> ()  [unwired: 1 out]
    n5 = local read "is publish loop stoped?"() -> (w23:bool)
    n6 = call "publish -- get frequency and voltage.vi"("publisher action"=publisher_action."set", "gamma IN (Hz)"=w24, "Voltage IN (V)"=w25, "freq IN (Hz)"=w26) -> ()  [unwired: 5 in, 3 out]
  }
  n7 = Unbundle By Name("pll monitor event pair IN") -> ("talkto event"=w3:refnum<user-event>)  [unwired: 1 out]
  n8 = Unbundle By Name("pll engine pair IN") -> ("talkto event"=w6:refnum<user-event>, "talkback event"=w5:refnum<user-event>)
  n9 = Create User Event(user event datatype=w11) -> (user event=w2:refnum<user-event>)  [unwired: 1 in, 1 out]
  n10 = Create User Event(user event datatype=w13) -> (user event=w1:refnum<user-event>)  [unwired: 1 in, 1 out]
  n11 = Create User Event(user event datatype=w9) -> (user event=w8:refnum<user-event>)  [unwired: 1 in, 1 out]
  n12 = register-events(w5, w8) -> (reference out=w15:refnum<event-registration>)  [unwired: 2 in, 1 out]
  n13 = register-events(w1) -> (reference out=w21:refnum<event-registration>)  [unwired: 2 in, 1 out]
  n14 = register-events(w2, w3) -> (reference out=w10:refnum<event-registration>)  [unwired: 2 in, 1 out]
  n15 = call "aggregator - vii - real - atomic.vi"("aggregator action"=agregator_--_action."empty!", "requested size"=100, "state IN"=T9 {"requested size"=20, "Array"=[], "actual number of elements"=0}) -> ("state OUT"=w16:T9)  [unwired: 5 in, 3 out]
  n16 = control-ref of="Plot: complex- hist"() -> (w17:refnum<vi>)
  n17 = control-ref of="Plot: complex plane"() -> (w14:refnum<vi>)
  n18 = while "communication Loop" {
    shift-right: [w32] -> _
    shift-left: w16 -> [w35]
    shift-right: [w33] -> _
    shift-left: w16 -> [w34]
    tunnel: w15 -> [w31]
    tunnel: w2 -> [w30]
    stop <- w29 stop-if-true
    n19 = event shown="[0] <talkback event>: User Event" {
      selector: w31 -> [_ _]
      dyn-events: _ -> [_ _]
      timeout: _ -> [_ _]
      tunnel: w35 -> [w41 w94]
      tunnel: w34 -> [w40 w93]
      tunnel: [w39 w93] -> w33
      tunnel: [w38 w94] -> w32
      tunnel: w30 -> [w36 _]
      tunnel: [_ w95] -> w29
      event User Event {
        n20 = event-data() -> ("message"=w37:enum16{"new", "void"})  [unwired: 1 in]
        n21 = case shown="\"new\"" w37 {
          tunnel: w41 -> [w43 w85]
          tunnel: w40 -> [w42 w82]
          tunnel: [w42 w81] -> w39
          tunnel: [w43 w52] -> w38
          tunnel: w36 -> [_ w45]
          frame "void", Default {
          }
          frame "new" {
            n22 = local read "plot hist time (sec)"() -> (w46:dbl)
            n23 = local read "dt (sec)"() -> (w47:dbl)
            n24 = local read "lorentzian"() -> (w48:T2)
            n25 = Divide(x=w46, y=w47) -> (x/y=w76:dbl)
            n26 = disable-structure shown="Enabled" {
              disable-tunnel: [w90 w92] -> w86
              disable-tunnel: w48 -> [w88 w91]
              disable-tunnel: [w87 w91] -> w50
              frame Disabled {
                n27 = call "lorentzian transformations.vi"("4 corner circle transformation"=four-corner_circle_transformation."get4corners", "lorentzian in"=w88) -> ("lorentzian out"=w87:T2, "4corners our"=w90:T3)  [unwired: 6 in, 2 out]
              }
              frame Enabled {
                n28 = Unbundle By Name(w91) -> ("4corners"=w92:T3)
              }
            }
            n29 = Round To Nearest(number=w76) -> (nearest integer value=w75:dbl)
            n30 = To Long Integer(number=w75) -> (32bit integer=w74:i32)
            n31 = call "aggregator - vii - complex - atomic.vi"("aggregator action"=agregator_--_action."append", "requested size"=w74, "state IN"=w85) -> ("state OUT"=w52:T13)  [unwired: 5 in, 3 out]
            n32 = Generate User Event(user event=w45, event data cluster="action: new" ("event data")) -> ()  [unwired: 2 in, 2 out]
            n33 = call "aggregator - vii - real - atomic.vi"("aggregator action"=agregator_--_action."append", "requested size"=w74, "state IN"=w82) -> ("state OUT"=w81:T9)  [unwired: 5 in, 3 out]
            n34 = call "draw complex lorentzian.vi"("4 corners"=w86) -> ("fancy circles"=→"Plot: complex plane":cluster{dbl[], dbl[]}[])  [unwired: 10 in]
            n35 = Unbundle By Name(w81) -> ("Array"=w68:dbl[])
            n36 = Unbundle By Name(w52) -> ("Array"=w69:cdb[])
            n37 = call "linear interp iiii- complex - z-omega.vi"("z"=w69, "omega"=w68) -> ("slope"=w67:cdb)  [unwired: 5 in, 8 out]
            n38 = Unbundle By Name(w50) -> ("4corners.z center"=w49:cdb, "A (VHz)"=w62:dbl, "G (Hz)"=w64:dbl)
            n39 = Complex To Polar(r * e^(i*theta)=w67) -> (r=w66:dbl)  [unwired: 1 out]
            n40 = Divide(x=w67, y=w66) -> (x/y=w65:cdb)
            n41 = call "lorentzian transformations.vi"("4 corner circle transformation"=four-corner_circle_transformation."get4corners", "lorentzian in"="lorentzian -- hist") -> ("4corners our"=w73:T3)  [unwired: 6 in, 3 out]
            n42 = Reciprocal(x=w64) -> (1/x=w63:dbl)
            n43 = Complex To Re/Im(x + iy=w69) -> (x=w79:dbl[], y=w78:dbl[])
            n44 = Compound Arithmetic op=MULTIPLY(w65, w63, w62, 1.1 ("value")) -> (w55:cdb)
            n45 = call "draw complex lorentzian.vi"("4 corners"=w73) -> ("fancy circles"=w71:cluster{dbl[], dbl[]}[])  [unwired: 10 in]
            n46 = Bundle(w79, w78) -> (w80:cluster{dbl[], dbl[]})  [unwired: 1 in]
            n47 = Add(x=w49, y=w55) -> (x+y=w61:cdb)
            n48 = Subtract(x=w49, y=w55) -> (x-y=w60:cdb)
            n49 = Complex To Re/Im(x + iy=w61) -> (x=w59:dbl, y=w57:dbl)
            n50 = Complex To Re/Im(x + iy=w60) -> (x=w58:dbl, y=w56:dbl)
            n51 = call "draw a line.vi"("y1"=w56, "y0"=w57, "x1"=w58, "x0"=w59) -> ("output cluster"=w53:cluster{dbl[], dbl[]})  [unwired: 7 in]
            n52 = Build Array (concatenate)(w80, w71, w53) -> (→"Plot: complex- hist":cluster{dbl[], dbl[]}[])
          }
        }
      }
      event User Event {
        n53 = event-data() -> ("communication"=w96:string)  [unwired: 1 in]
        n54 = case shown="\"communication: exit\"" w96 {
          tunnel: [_ TRUE] -> w95
          frame "void", Default {
          }
          frame "communication: exit" {
          }
        }
      }
    }
  }
  n55 = while "interface Loop" {
    tunnel: w21 -> [w105]
    tunnel: w1 -> [w104]
    tunnel: w14 -> [w103]
    tunnel: w17 -> [w102]
    tunnel: w6 -> [w101]
    tunnel: w2 -> [w99]
    tunnel: w8 -> [w98]
    stop <- w100 stop-if-true
    n56 = event shown="[7] Key Down" {
      selector: w105 -> [_ _ _ _ _ _ _ _]
      dyn-events: _ -> [_ _ _ _ _ _ _ _]
      timeout: _ -> [_ _ _ _ _ _ _ _]
      tunnel: [_ "Toggle PLL :@" _ "Reset freq :r" "Reset lore :q" "reset from basic" "save lor for later" _] -> _
      tunnel: w104 -> [w110 w164 _ w199 w202 _ _ w213]
      tunnel: w103 -> [w111 _ w170 _ _ _ _ w212]
      tunnel: w102 -> [_ _ _ _ _ _ _ w211]
      tunnel: w101 -> [w109 _ _ _ _ _ _ _]
      tunnel: [w108 _ _ _ _ _ _ _] -> w100
      tunnel: w99 -> [w107 _ _ _ _ _ _ _]
      tunnel: w98 -> [w106 _ _ _ _ _ _ _]
      event User Event {
        n57 = event-data() -> ("interface"=w112:T8)  [unwired: 1 in]
        n58 = case shown="\"pause pll\"" w112 {
          tunnel: w111 -> [_ _ _ _ _ _ _ _ w156 _]
          tunnel: w110 -> [_ _ w117 _ _ _ _ w140 _ w158]
          tunnel: w109 -> [_ w114 w122 w125 w128 w129 _ _ _ _]
          tunnel: [_ _ _ _ _ _ TRUE _ _ _] -> w108
          tunnel: w107 -> [_ _ _ _ _ _ w134 _ _ _]
          tunnel: w106 -> [_ _ _ _ _ _ w131 _ _ _]
          frame "void", Default {
          }
          frame "accept frequency" {
            n59 = Generate User Event(user event=w114, event data cluster=T14 {"message"=enum."reset"} ("event data")) -> ()  [unwired: 2 in, 2 out]
          }
          frame "accept lorentzian" {
            n60 = Generate User Event(user event=w117, event data cluster=pll_internal_user_event_action."update cursors" ("event data")) -> ()  [unwired: 2 in, 2 out]
            n61 = call "publish -- lorentzian.vi"("publisher action"=publisher_action."get") -> ("lorentzian OUT"=w121:T2)  [unwired: 10 in]
            n62 = Generate User Event(user event=w122, event data cluster=T14 {"message"=enum."update request"} ("event data")) -> ()  [unwired: 2 in, 2 out]
            n63 = call "lorentzian transformations.vi"("4 corner circle transformation"=four-corner_circle_transformation."get4corners", "lorentzian in"=w121) -> ("lorentzian out"=w120:T2)  [unwired: 6 in, 3 out]
            n64 = local write "lorentzian"(w120) -> ()
            n65 = local write "lorentzian -- hist"(w120) -> ()
          }
          frame "pause pll" {
            n66 = Generate User Event(user event=w125, event data cluster=T14 {"message"=enum."pause"} ("event data")) -> ()  [unwired: 2 in, 2 out]
            n67 = local write "PLL is ON"(FALSE ("PLL ON")) -> ()
          }
          frame "unpause pll" {
            n68 = Generate User Event(user event=w128, event data cluster=T14 {"message"=enum."unpause"} ("event data")) -> ()  [unwired: 2 in, 2 out]
            n69 = local write "PLL is ON"(TRUE ("PLL ON")) -> ()
          }
          frame "start pll async" {
            n70 = Generate User Event(user event=w129, event data cluster=T14 {"message"=enum."start"} ("event data")) -> ()  [unwired: 2 in, 2 out]
          }
          frame "exit" {
            n71 = Generate User Event(user event=w134, event data cluster="action: exit" ("event data")) -> ()  [unwired: 2 in, 2 out]
            n72 = Generate User Event(user event=w131, event data cluster="communication: exit" ("event data")) -> ()  [unwired: 2 in, 2 out]
            n73 = local write "PLL is ON"(FALSE ("PLL ON")) -> ()
            n74 = local write "is publish loop stoped?"(TRUE ("Stoped?")) -> ()
          }
          frame "toggle pll async" {
            n75 = local read "PLL is ON"() -> (w139:bool)
            n76 = case shown="True" w139 {
              tunnel: [pll_internal_user_event_action."unpause pll" ("event data") pll_internal_user_event_action."pause pll" ("event data")] -> w138
              frame False {
              }
              frame True {
              }
            }
            n77 = Generate User Event(user event=w140, event data cluster=w138) -> ()  [unwired: 2 in, 2 out]
          }
          frame "update cursors" {
            n78 = local read "lorentzian"() -> (w143:T2)
            n79 = Unbundle By Name(w143) -> ("4corners.z(inf)"=w151:cdb, "4corners.z(0)"=w144:cdb)
            n80 = Complex To Re/Im(x + iy=w151) -> (x=w153:dbl, y=w152:dbl)
            n81 = Complex To Re/Im(x + iy=w144) -> (x=w147:dbl, y=w146:dbl)
            n82 = call "replace cursor - plot ref - V2.vi"("Plot ref in"=w156, "new X"=w153, "new  Y"=w152, "cursor index"=2, "cursor action"=cursor_action."write", "Color Box"=u32 16746738) -> ()  [unwired: 10 in, 4 out]
            n83 = call "replace cursor - plot ref - V2.vi"("Plot ref in"=w156, "new X"=w147, "new  Y"=w146, "cursor index"=3, "cursor action"=cursor_action."write", "Color Box"=u32 10682154) -> ()  [unwired: 10 in, 4 out]
          }
          frame "toggle sweeper" {
            n84 = case shown="True" "PLL is ON" {
              tunnel: w158 -> [_ w160]
              frame False {
              }
              frame True {
                n85 = Generate User Event(user event=w160, event data cluster=pll_internal_user_event_action."pause pll" ("event data")) -> ()  [unwired: 2 in, 2 out]
              }
            }
            n86 = Generate User Event(user event=w158, event data cluster=pll_internal_user_event_action."start sweeper" ("event data")) -> ()  [unwired: 2 in, 2 out]
          }
        }
      }
      event "Toggle PLL :@": Value Change {
        w162 = pll_internal_user_event_action."toggle pll async"  # event data
        n87 = event-data() -> ()  [unwired: 1 in, 1 out]
        n88 = Generate User Event(user event=w164, event data cluster=w162) -> ()  [unwired: 2 in, 2 out]
      }
      event "Plot: complex plane": Cursor Move {
        n89 = event-data() -> ("CursIdx"=w169:i32)  [unwired: 1 in]
        n90 = local read "lorentzian"() -> (w168:T2)
        n91 = case shown="2" w169 {
          selector: w169 -> [_ w182 w192]
          tunnel: w170 -> [_ w176 w191]
          tunnel: w168 -> [w171 w172 w190]
          tunnel: [w171 w173 w187] -> w166
          frame 0, Default {
          }
          frame 2 {
            n92 = call "replace cursor - plot ref - V2.vi"("Plot ref in"=w176, "cursor index"=w182, "cursor action"=cursor_action."read") -> ("read X"=w184:dbl, "read Y"=w185:dbl)  [unwired: 13 in, 2 out]
            n93 = Re/Im To Complex(1:w185, 2:w184) -> (0:w183:cdb)
            n94 = Bundle By Name(cluster=w172, "bg (V)"=w183) -> (w181:T2)
            n95 = call "lorentzian transformations.vi"("4 corner circle transformation"=four-corner_circle_transformation."get4corners", "lorentzian in"=w181) -> ("lorentzian out"=w173:T2)  [unwired: 6 in, 3 out]
            n96 = Unbundle By Name(w173) -> ("4corners.z(0)"=w179:cdb)
            n97 = Complex To Re/Im(x + iy=w179) -> (x=w178:dbl, y=w177:dbl)
            n98 = call "replace cursor - plot ref - V2.vi"("Plot ref in"=w176, "new X"=w178, "new  Y"=w177, "cursor index"=3, "cursor action"=cursor_action."write") -> ()  [unwired: 11 in, 4 out]
          }
          frame 3 {
            n99 = call "replace cursor - plot ref - V2.vi"("Plot ref in"=w191, "cursor index"=w192, "cursor action"=cursor_action."read") -> ("read X"=w194:dbl, "read Y"=w195:dbl)  [unwired: 13 in, 2 out]
            n100 = Re/Im To Complex(1:w195, 2:w194) -> (0:w193:cdb)
            n101 = Bundle By Name(cluster=w190, "4corners.z(0)"=w193) -> (w189:T2)
            n102 = call "lorentzian transformations.vi"("4 corner circle transformation"=four-corner_circle_transformation."update lorentzian -- from z0", "lorentzian in"=w189) -> ("lorentzian out"=w187:T2)  [unwired: 6 in, 3 out]
          }
        }
        n103 = call "lorentzian transformations.vi"("4 corner circle transformation"=four-corner_circle_transformation."get4corners", "lorentzian in"=w166) -> ("lorentzian out"=w165:T2)  [unwired: 6 in, 3 out]
        n104 = local write "lorentzian"(w165) -> ()
      }
      event "Reset freq :r": Value Change {
        n105 = event-data() -> ()  [unwired: 1 in, 1 out]
        n106 = Generate User Event(user event=w199, event data cluster=pll_internal_user_event_action."accept frequency" ("event data")) -> ()  [unwired: 2 in, 2 out]
      }
      event "Reset lore :q": Value Change {
        n107 = event-data() -> ()  [unwired: 1 in, 6 out]
        n108 = Generate User Event(user event=w202, event data cluster=pll_internal_user_event_action."accept lorentzian" ("event data")) -> ()  [unwired: 2 in, 2 out]
      }
      event "reset from basic": Value Change {
        n109 = event-data() -> ()  [unwired: 1 in, 6 out]
        n110 = local read "lorentzian -- basic"() -> (w204:T2)
        n111 = call "lorentzian transformations.vi"("4 corner circle transformation"=four-corner_circle_transformation."get4corners", "lorentzian in"=w204) -> ("lorentzian out"=w203:T2)  [unwired: 6 in, 3 out]
        n112 = local write "lorentzian"(w203) -> ()
      }
      event "save lor for later": Value Change {
        n113 = event-data() -> ()  [unwired: 1 in, 6 out]
        n114 = local read "lorentzian"() -> (w208:T2)
        n115 = call "lorentzian transformations.vi"("4 corner circle transformation"=four-corner_circle_transformation."get4corners", "lorentzian in"=w208) -> ("lorentzian out"=w207:T2)  [unwired: 6 in, 3 out]
        n116 = local write "lorentzian -- basic"(w207) -> ()
      }
      event Key Down {
        n117 = event-data() -> ("Char"=w215:i16, "VKey"=w217:T4)  [unwired: 1 in]
        "Char" <- w215
        "VKey" <- w217
        n118 = Build Array(w215) -> (w216:i16[])
        n119 = Byte Array To String(unsigned byte array=w216) -> (string=w214:string)
        n120 = case shown="\"Up\"..\"Right\"" w217 {
          selector: w217 -> [_ _ _ _ w242]
          tunnel: w215 -> [_ _ _ _ _]
          tunnel: w214 -> [w221 _ _ _ _]
          tunnel: w213 -> [w220 _ _ _ _]
          tunnel: w212 -> [w219 _ _ _ w241]
          tunnel: w211 -> [w218 _ _ _ w240]
          frame "ASCII", Default {
            n121 = case shown="\"r\"" w221 {
              selector: w221 -> [_ w224 _ _ _ _ _]
              tunnel: w220 -> [_ _ w232 _ w234 w236 w238]
              tunnel: w219 -> [_ w223 _ _ _ _ _]
              tunnel: w218 -> [_ w222 _ _ _ _ _]
              frame "0", Default {
              }
              frame "<", ">", "?", "A", "z" {
                n122 = case shown="\"A\"" w224 {
                  tunnel: [cursor_action."zoom out 20%" ("cursor action") cursor_action."zoom in 20%" ("cursor action") cursor_action."smart zoom out&aspect" ("cursor action") cursor_action."smart zoom out" ("cursor action") cursor_action."zoom to aspect ratio 1" ("cursor action")] -> w225
                  frame ">" {
                  }
                  frame "<" {
                  }
                  frame "?" {
                  }
                  frame "A" {
                  }
                  frame "z", Default {
                  }
                }
                n123 = call "replace cursor - plot ref - V2.vi"("Plot ref in"=w223, "cursor action"=w225) -> ()  [unwired: 14 in, 4 out]
                n124 = call "replace cursor - plot ref - V2.vi"("Plot ref in"=w222, "cursor action"=w225) -> ()  [unwired: 14 in, 4 out]
              }
              frame "r" {
                (unwired) "reset frequency" ("event data")
                n125 = Generate User Event(user event=w232, event data cluster=pll_internal_user_event_action."accept frequency" ("event data")) -> ()  [unwired: 2 in, 2 out]
              }
              frame "'", ";", "[", "]", "{", "}" {
              }
              frame "@" {
                (unwired) "toggle PLL" ("event data")
                n126 = Generate User Event(user event=w234, event data cluster=pll_internal_user_event_action."toggle pll async" ("event data")) -> ()  [unwired: 2 in, 2 out]
              }
              frame "#" {
                (unwired) "(sweeper) sweep!" ("event data")
                n127 = Generate User Event(user event=w236, event data cluster=pll_internal_user_event_action."toggle sweeper" ("event data")) -> ()  [unwired: 2 in, 2 out]
              }
              frame "q" {
                (unwired) "reset lorentzian" ("event data")
                n128 = Generate User Event(user event=w238, event data cluster=pll_internal_user_event_action."accept lorentzian" ("event data")) -> ()  [unwired: 2 in, 2 out]
              }
            }
          }
          frame "Escape" {
          }
          frame "PageUp" {
          }
          frame "PageDown" {
          }
          frame "Up".."Right" {
            n129 = case shown="\"Down\"" w242 {
              tunnel: [cursor_action."move range right 20%" ("cursor action") cursor_action."move range left 20%" ("cursor action") cursor_action."move range up 20%" ("cursor action") cursor_action."move range down 20%" ("cursor action")] -> w239
              frame "Right", Default {
              }
              frame "Left" {
              }
              frame "Up" {
              }
              frame "Down" {
              }
            }
            n130 = call "replace cursor - plot ref - V2.vi"("Plot ref in"=w240, "cursor action"=w239) -> ()  [unwired: 14 in, 4 out]
            n131 = call "replace cursor - plot ref - V2.vi"("Plot ref in"=w241, "cursor action"=w239) -> ()  [unwired: 14 in, 4 out]
          }
        }
      }
    }
  }
  n132 = while "action Loop" {
    tunnel: w10 -> [w250]
    tunnel: w2 -> [w248]
    tunnel: w1 -> [w247]
    stop <- w249 stop-if-true
    n133 = event shown="[1] <talkto event>: User Event" {
      selector: w250 -> [_ _]
      dyn-events: _ -> [_ _]
      timeout: _ -> [_ _]
      tunnel: [w252 _] -> w249
      tunnel: w248 -> [_ w276]
      tunnel: w247 -> [w251 w275]
      event User Event {
        n134 = event-data() -> ("action"=w253:string)  [unwired: 1 in]
        n135 = case shown="\"action: new\", Default" w253 {
          tunnel: [_ TRUE] -> w252
          tunnel: w251 -> [_ _]
          frame "action: new", Default {
            w261 = 0.0 ("new X")
            n136 = call "publish -- pll result.vi"("publisher action"=publisher_action."get") -> ("pll result OUT"=w269:T16)  [unwired: 10 in]
            n137 = Unbundle By Name(w269) -> ("freq (Hz)"=w270:dbl, "gamma (Hz)"=w271:dbl, "Voltage (V)"=w272:cdb)
            "f (Hz)" <- w270
            "G (Hz)" <- w271
            n138 = control-ref of="Plot: complex plane"() -> (w273:refnum<vi>)
            n139 = Bundle By Name(cluster=T5 {"freq (Hz)"=0.0, "gamma (Hz)"=0.0, "Voltage (V)"=0.0+0.0i} ("publish message"), "freq (Hz)"=w270, "gamma (Hz)"=w271, "Voltage (V)"=w272) -> (→"publish message":T5)
            n140 = Complex To Re/Im(x + iy=w272) -> (x=→"zi out Re (V)":dbl, y=→"zi out Im (V)":dbl)
            n141 = Complex To Re/Im(x + iy=w272) -> (x=w265:dbl, y=w264:dbl)
            n142 = call "replace cursor - plot ref - V2.vi"("Plot ref in"=w273, "new X"=w265, "new  Y"=w264, "cursor index"=0, "cursor action"=cursor_action."write", "Color Box"=u32 327424) -> ("Plot ref out"=w263:refnum<vi>)  [unwired: 10 in, 3 out]
            n143 = call "replace cursor - plot ref - V2.vi"("Plot ref in"=w263, "new X"=w261, "new  Y"=w261, "cursor index"=1, "cursor action"=cursor_action."write", "Color Box"=u32 5880319) -> ()  [unwired: 10 in, 4 out]
          }
          frame "action: exit" {
          }
        }
      }
      event User Event {
        (unwired) T17."stop" ("message")
        n144 = event-data() -> ("message"=w277:T17)  [unwired: 1 in]
        n145 = case shown="\"exit\"" w277 {
          tunnel: w276 -> [_ _]
          tunnel: w275 -> [_ w278]
          frame "stop", Default {
          }
          frame "exit" {
            n146 = Generate User Event(user event=w278, event data cluster=pll_internal_user_event_action."exit" ("event data")) -> ()  [unwired: 2 in, 2 out]
          }
        }
      }
    }
  }
  "is publish loop stoped?" <- FALSE ("Stoped?")
